vi "send error message.vi"(8 "error in":errorcluster, 10 "error to send":errorcluster, 11 "message queue in":T1) -> (0 "error out":errorcluster, 3 "message queue out":T1)   [LabVIEW 2013, in "DCAF Execution Service.lvlib"]
uses:
  DCAF Execution Service.lvlib
  <vilib>/NI/AMC/Message Queue.ctl
  <vilib>/NI/AMC/Message.ctl
  <vilib>/NI/Tools/Keyed Array/KeyedArray.ctl
  common reponses to network process.ctl
  <vilib>/NI/AMC/Create Single Message.vi
  <vilib>/NI/AMC/Update Message Routing Info.vi
  <vilib>/NI/AMC/Send Message.vi
  <vilib>/NI/AMC/AMC.lvlib
  <vilib>/NI/Tools/Keyed Array/Tools_KeyedArray.lvlib
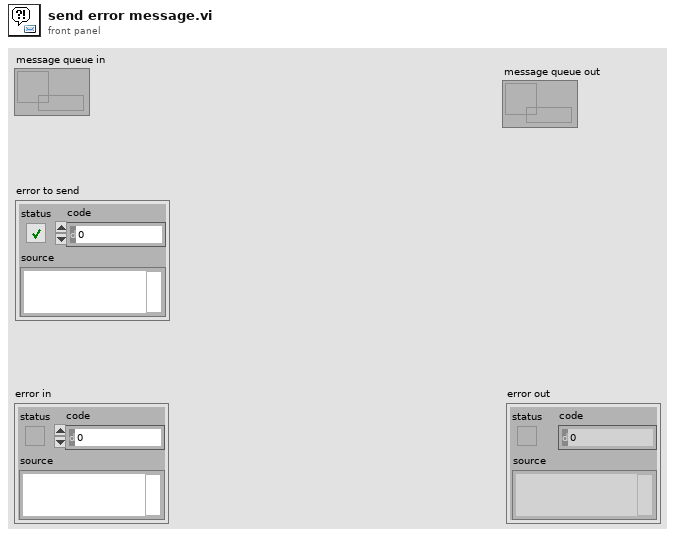
[diagram p1: front panel]
types:
  T1 = typedef "AMC.lvlib/Message Queue.ctl" = refnum<queue>
  T2 = typedef "DCAF Execution Service.lvlib/common reponses to network process.ctl" = enum16{"System Error", "Load Report", "Action Response", "Engine Status"}
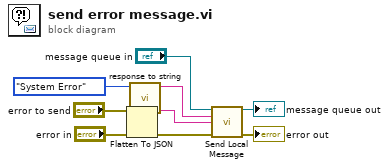
[diagram p0: block diagram]
diagram:
  n1 = Flatten To JSON(anything="error to send", error in (no error)="error in") -> (JSON string=w3:string, 11:w4:errorcluster)  [unwired: 1 in]
  n2 = call "response to string.vi"("responses"=common_reponses_to_network_process."System Error") -> ("command string"=w2:string)  [unwired: 10 in]
  n3 = call <vilib>:"Send Local Message.vi"("message queue in"="message queue in", "message name"=w2, "message value"=w3, "error in"=w4) -> ("message queue out"=→"message queue out":T1, "error out"=→"error out":errorcluster)  [unwired: 9 in, 1 out]
